vi "Curtin1_DAQFiles.vi"(9 "Settings":T2={"Name of test"="", "Date"=timestamp(0 s since 1904-01-01), "Location"="", "Template"="", "Soundcard"="OCTA-CAPTURE", "resolution"=32, "Sampling rate"=48000, "Ch1 Gain "=10.0, "Ch2 Gain"=20.0, "Sample time (s)"=0.3, "Pre-trigger (s)"=0.001, "Hammer Threshold"=0.01, "Positions"=12, "Taps/Position"=5, "Set Names"="H,V", "Freq resolution"=1.0, "Hammer cutoff"=0.025, "Mic cutoff"=0.25, "Double bounce "=0.01, "Hammer Cal"=1.0, "dB Offset"=0.0, "Accel Cal"=1.0, "Vibrometer Cal"=1.0, "Mic Cal"=49.38, "Output"=2, "Voltage Cal"=13.8, "Vibrometer Port"="ASRL27::INSTR", "Range"=4, "High Pass"=2, "Bandwidth"=4, "X Range"=[], "Y Range"=[], "dB Spread"=0.0, "Trigger"=0, "Ch_1"=25, "Ch_2"=25, "flip?"=FALSE, "60Hz"=FALSE, "Time offset"=0.0, "Piezo Cal"=1.0, "Default Notes"=""} {"Ch_2" min=1 step=1; "Ch_1" min=1 max=100 step=1; "Trigger" items=["Hammer (force)", "Self-tap", "Spacebar"]; "Bandwidth" items=["1 kHz"=1, "5 kHz"=5, "10 kHz"=10, "25 kHz"=25, "50 kHz"=50, "100 kHz"=100]; "High Pass" items=["Off", "13 Hz", "104 Hz"]; "Range" items=["10 mm/s"=1, "20 mm/s"=2, "50 mm/s"=5, "100 mm/s"=10, "200 mm/s"=20, "500 mm/s"=50, "1 m/s"=100, "2 m/s"=200]; "Output" items=["Accelerometer", "Speed (from acceleration)", "Microphone", "Vibrometer", "Piezo"]; "Voltage Cal" format="%#_13g"; "Ch2 Gain" format="%#_13g"; "Ch1 Gain" format="%#_13g"; "Double bounce" min=0.0; "Mic cutoff" min=0.0 format="%#_4g"; "Hammer cutoff" min=0.0 format="%#_4g"; "Freq resolution" min=0.0; "Pre-trigger (s)" format="%#_13g"; "Date" format="%<%H:%M\n%d/%m/%y>T"; "resolution" items=["16 bit"=16, "24 bit"=24, "32 bit"=32]; "Sampling rate" items=["22050 samp/s"=22050, "44100 samp/s"=44100, "48000 samp/s"=48000]}, 11 "Files in":T3[](array[typedef])) -> (3 "Files out":T3[](array[typedef]))   [LabVIEW 2022 SP3]
uses:
  Curtin1_Label.ctl
  PreferencesControl.ctl
  <vilib>/Utility/error.llb/Trim Whitespace One-Sided.vi
  Mic/Mic_Global.vi
panel:
  in  "delete":bool
  in  "OK Button":bool
  in  "Autoload":T1(ring)=enum."Entire Run"
  out "filenames":string[](array[string])
  # "Hz"
  # "dB"
  # "dB"
  # "sec"
  # "sec"
  # "mV/Pa"
  # "mV/m/s2"
  # "mV/mm/s"
  # "V/N"
  # "sec"
  # "sec"
  # "mV/N"
  # "a.u."
  # "a.u."
  # "sec"
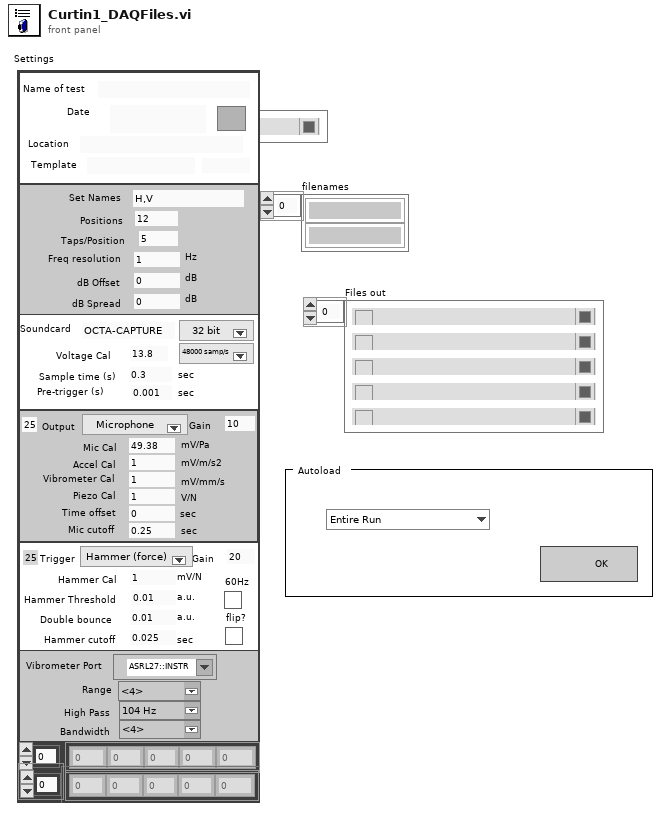
[diagram p1: front panel]
types:
  T1 = enum16{"Nothing", "Entire Run", "All Sets", "All Positions", "All Taps"}
  T2 = typedef "PreferencesControl.ctl" = cluster{"Name of test":string, "Date":timestamp, "Location":string, "Template":string, "Soundcard":string, "resolution":u16, "Sampling rate":u16, "Ch1 Gain ":dbl, "Ch2 Gain":dbl, "Sample time (s)":dbl, "Pre-trigger (s)":dbl, "Hammer Threshold":dbl, "Positions":i16, "Taps/Position":i16, "Set Names":string, "Freq resolution":dbl, "Hammer cutoff":dbl, "Mic cutoff":dbl, "Double bounce ":dbl, "Hammer Cal":dbl, "dB Offset":dbl, "Accel Cal":dbl, "Vibrometer Cal":dbl, "Mic Cal":dbl, "Output":u16, "Voltage Cal":dbl, "Vibrometer Port":refnum<visa-resource-name>, "Range":u16, "High Pass":u16, "Bandwidth":u16, "X Range":cluster{"Minimum":dbl, "Maximum":dbl, "Increment":dbl, "Minor Increment":dbl, "Start":dbl}[], "Y Range":cluster{"Minimum":dbl, "Maximum":dbl, "Increment":dbl, "Minor Increment":dbl, "Start":dbl}[], "dB Spread":dbl, "Trigger":u16, "Ch_1":u8, "Ch_2":u8, "flip?":bool, "60Hz":bool, "Time offset":dbl, "Piezo Cal":dbl, "Default Notes":string}
  T3 = typedef "Curtin1_Label.ctl" = cluster{"Show?":bool, "Name":string, "Color":u32, "Path":path, "Show Notes":bool}
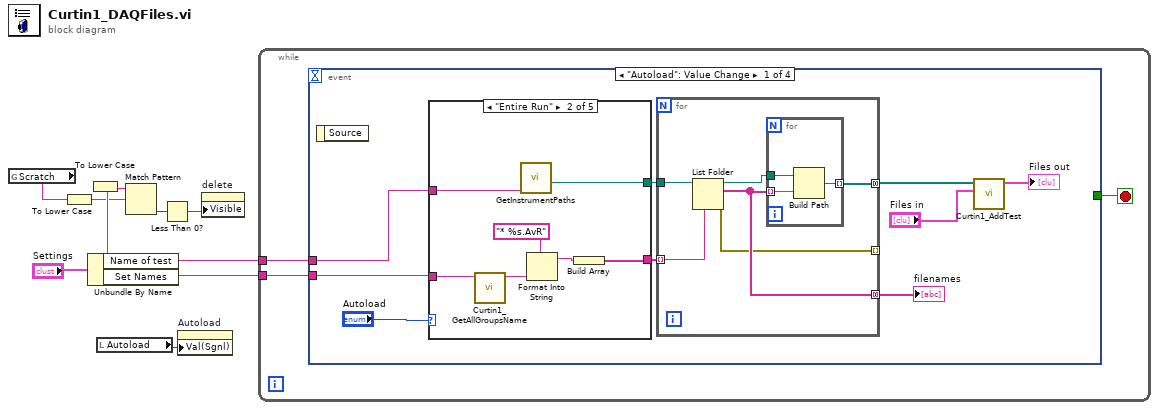
[diagram p0: block diagram]
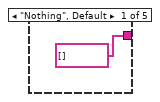
[diagram p2: hidden frame]
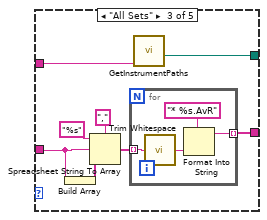
[diagram p3: hidden frame]
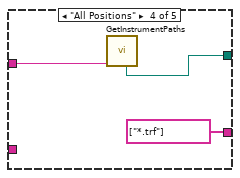
[diagram p4: hidden frame]
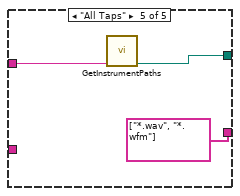
[diagram p5: hidden frame]
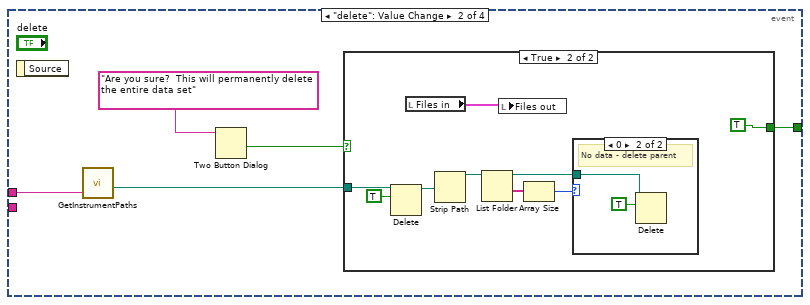
[diagram p6: hidden frame]
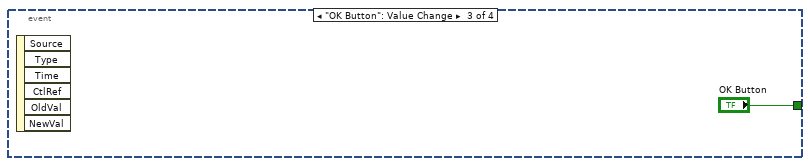
[diagram p9: hidden frame]
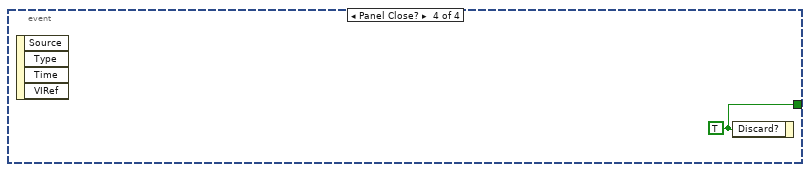
[diagram p10: hidden frame]
diagram:
  n1 = global read "Mic_Global.vi" "Scratch"() -> (w3:string)
  n2 = To Lower Case(string=w3) -> (all lower case string=w2:string)
  n3 = Unbundle By Name("Settings") -> ("Name of test"=w4:string, "Set Names"=w7:string)
  n4 = To Lower Case(string=w4) -> (all lower case string=w1:string)
  n5 = local read "Autoload"() -> (w9:T1)
  n6 = Match Pattern(string=w1, regular expression=w2) -> (offset past match=w6:i32)  [unwired: 1 in, 3 out]
  n7 = Less Than 0?(x=w6) -> (x < 0?=w5:bool)
  n8 = property on="Autoload" class="Enum (strict)"("Val(Sgnl)"=w9) -> ()  [unwired: 2 in, 2 out]
  n9 = property on="delete" class="Bool"("Visible"=w5) -> ()  [unwired: 2 in, 2 out]
  n10 = while {
    tunnel: w4 -> [w11]
    tunnel: w7 -> [w10]
    stop <- w12 stop-if-true
    n11 = event shown="[0] \"Autoload\": Value Change" {
      selector: _ -> [_ _ _ _]
      dyn-events: _ -> [_ _ _ _]
      timeout: _ -> [_ _ _ _]
      tunnel: [_ w59 "OK Button" w74] -> w12
      tunnel: w11 -> [w13 w58 _ _]
      tunnel: w10 -> [w14 _ _ _]
      event "Autoload": Value Change {
        n12 = event-data() -> ()  [unwired: 1 in, 1 out]
        n13 = case shown="\"Entire Run\"" "Autoload" {
          tunnel: w14 -> [_ w36 w46 _ _]
          tunnel: [string[] [] w34 w41 string[] ["*.trf"] string[] ["*.wav", "*.wfm"]] -> w18
          tunnel: w13 -> [_ w33 w39 w53 w56]
          tunnel: [_ w32 w40 w52 w54] -> w15
          frame "Nothing", Default {
          }
          frame "Entire Run" {
            n14 = call "Curtin1_GetAllGroupsName.vi"("Set Names in"=w36) -> ("Set Names out"=w38:string)  [unwired: 10 in]
            n15 = call "GetInstrumentPaths.vi"("Instrument"=w33) -> ("Path To Test Folder"=w32:path)  [unwired: 6 in, 4 out]
            n16 = Format Into String(format string="* %s.AvR" ("pattern"), w38) -> (resulting string=w35:string)  [unwired: 2 in, 1 out]
            n17 = Build Array(w35) -> (w34:string[])
          }
          frame "All Sets" {
            n18 = Build Array(w46) -> (w45:string[])
            n19 = Spreadsheet String To Array(delimiter (Tab)=",", format string="%s", spreadsheet string=w46, array type (2D Dbl)=w45) -> (array=w42:string[])
            n20 = for {
              tunnel: w42 -> [w49] mode=indexing
              tunnel: [w48] -> w41 mode=indexing
              n21 = call <vilib>:"Trim Whitespace.vi"("string"=w49) -> ("trimmed string"=w47:string)  [unwired: 1 in]
              n22 = Format Into String(format string="* %s.AvR" ("pattern"), w47) -> (resulting string=w48:string)  [unwired: 2 in, 1 out]
            }
            n23 = call "GetInstrumentPaths.vi"("Instrument"=w39) -> ("Path To Test Folder"=w40:path)  [unwired: 6 in, 4 out]
          }
          frame "All Positions" {
            n24 = call "GetInstrumentPaths.vi"("Instrument"=w53) -> ("Path To TRF Folder"=w52:path)  [unwired: 6 in, 4 out]
          }
          frame "All Taps" {
            n25 = call "GetInstrumentPaths.vi"("Instrument"=w56) -> ("Path To Raw Folder"=w54:path)  [unwired: 6 in, 4 out]
          }
        }
        n26 = for {
          tunnel: [w26] -> w20 mode=concatenating
          tunnel: w18 -> [w25] mode=indexing
          tunnel: [w24] -> w16 mode=concatenating
          tunnel: [w23] -> _ mode=indexing
          tunnel: w15 -> [w22]
          n27 = List Folder(path=w22, pattern=w25) -> (path out=w27:path, filenames=w24:string[], error out=w23:errorcluster)  [unwired: 2 in, 1 out]
          n28 = for {
            tunnel: w24 -> [w30] mode=indexing
            tunnel: w27 -> [w29]
            tunnel: [w28] -> w26 mode=indexing
            n29 = Build Path(base path=w29, name or relative path=w30) -> (appended path=w28:path)
          }
        }
        "filenames" <- w16
        n30 = call "Curtin1_AddTest.vi"("Old Files"="Files in", "Selected Paths"=w20) -> ("New Files"=→"Files out":T3[])  [unwired: 9 in]
      }
      event "delete": Value Change {
        n31 = event-data() -> ()  [unwired: 1 in, 1 out]
        n32 = call "GetInstrumentPaths.vi"("Instrument"=w58) -> ("Path To Test Folder"=w57:path)  [unwired: 6 in, 4 out]
        n33 = Two Button Dialog(message="Are you sure?  This will permanently delete the entire data set") -> (T button?=w60:bool)  [unwired: 2 in]
        n34 = case shown="True" w60 {
          tunnel: [_ TRUE ("Discard?")] -> w59
          tunnel: w57 -> [_ w68]
          frame False {
          }
          frame True {
            n35 = Delete(path (use dialog)=w68, entire hierarchy (F)=TRUE) -> (deleted path=w66:path)  [unwired: 3 in, 2 out]
            n36 = local read "Files in"() -> (w70:T3[])
            n37 = Strip Path(path=w66) -> (stripped path=w65:path)  [unwired: 1 out]
            n38 = List Folder(path=w65) -> (path out=w62:path, folder names=w64:string[])  [unwired: 3 in, 2 out]
            n39 = local write "Files out"(w70) -> ()
            n40 = Array Size(array=w64) -> (size(s)=w63:i32)
            n41 = case shown="0" w63 {
              tunnel: w62 -> [_ w71]
              frame Default {
              }
              frame 0 {
                # "No data - delete parent"
                n42 = Delete(path (use dialog)=w71, entire hierarchy (F)=TRUE) -> ()  [unwired: 3 in, 3 out]
              }
            }
          }
        }
      }
      event "OK Button": Value Change {
        n43 = event-data() -> ()  [unwired: 1 in, 6 out]
      }
      event Panel Close? {
        w74 = TRUE ("Discard?")
        n44 = event-data() -> ()  [unwired: 1 in, 4 out]
        n45 = event-data("Discard?"=w74) -> ()  [unwired: 1 in, 1 out]
      }
    }
  }
